vi "Calc Arc Angles.vi"(10 "Arc CMD":T1={"N"=0.0, "GCODE"="", "X"=2.0396, "Y"=0.1665, "Z"=0.0, "E"=0.0, "I"=0.205, "J"=0.131, "S"=0.0, "F"=0.0}, 11 "Initial CMD":T1={"N"=0.0, "GCODE"="", "X"=1.6296, "Y"=0.1665, "Z"=-0.05, "E"=0.0, "I"=0.0, "J"=0.0, "S"=0.0, "F"=0.0}) -> (0 "travel angle out":dbl=114.84085989051317 format="%.5f", 2 "start angle (tangent)":dbl=212.57957005474344 format="%#_8g", 3 "R":dbl=0.2432817296880306 format="%#_9g")   [LabVIEW 2014]
uses:
  GCode Parser/GCode Command Cluster.ctl
panel:
  out "x*y":dbl=32.57957005474343
  out "V2Y":dbl=-0.13099999999999998
  out "V2X":dbl=0.20500000000000007
  out "V1Y":dbl=-0.13099999999999998
  out "V1X":dbl=-0.20500000000000007
  out "theta (degrees)":dbl=-114.84085989051317 format="%.2f"
  out "theta (radians)":dbl=-2.0043511209109495 format="%.3f"
  # "G01 X1.6296 Y0.1665 Z-0.0500\nG03 X2.0396 Y0.1665 I0.2050 J0.1310"
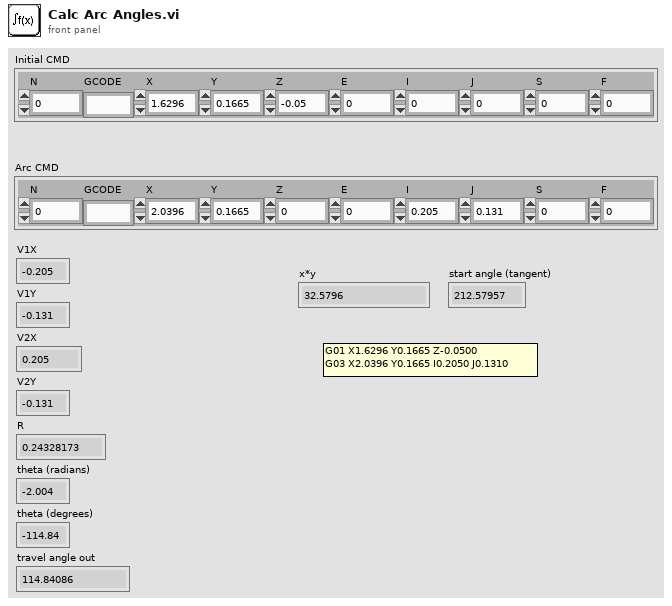
[diagram p1: front panel]
types:
  T1 = typedef "GCode Command Cluster.ctl" = cluster{"N":dbl, "GCODE":string, "X":dbl, "Y":dbl, "Z":dbl, "E":dbl, "I":dbl, "J":dbl, "S":dbl, "F":dbl}
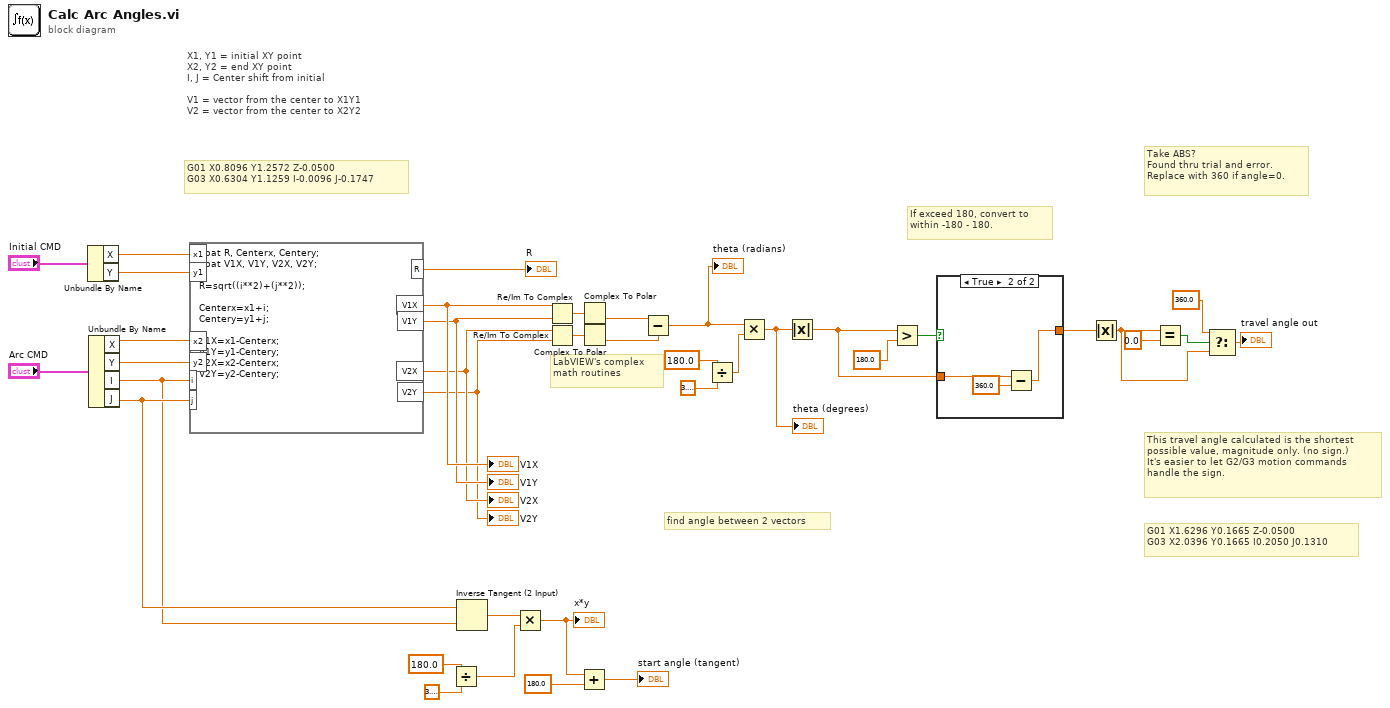
[diagram p0: block diagram]
diagram:
  # "This travel angle calculated is the shortest\npossible value, magnitude only. (no sign.)\nIt's easier to let G2/G3 motion commands\nhandle the sign."
  # "If exceed 180, convert to \nwithin -180 - 180."
  # "G01 X1.6296 Y0.1665 Z-0.0500\nG03 X2.0396 Y0.1665 I0.2050 J0.1310"
  # "Take ABS?\nFound thru trial and error.\nReplace with 360 if angle=0."
  # "find angle between 2 vectors"
  # "X1, Y1 = initial XY point\nX2, Y2 = end XY point\nI, J = Center shift from initial \n\nV1 = vector from the center to X1Y1\nV2 = vector from the center to X2Y2"
  # "LabVIEW's complex\nmath routines"
  # "G01 X0.8096 Y1.2572 Z-0.0500\nG03 X0.6304 Y1.1259 I-0.0096 J-0.1747"
  n1 = Unbundle By Name("Initial CMD") -> ("X"=w18:dbl, "Y"=w19:dbl)
  n2 = Unbundle By Name("Arc CMD") -> ("X"=w17:dbl, "Y"=w16:dbl, "I"=w14:dbl, "J"=w15:dbl)
  n3 = formula code="float R, Centerx, Centery;\nfloat V1X, V1Y, V2X, V2Y;\n\nR=sqrt((i**2)+(j**2));\n\nCenterx=x1+i;\nCentery=y1+j;\n\nV1X=x1-Centerx;\nV1Y=y1-Centery;\nV2X=x2-Centerx;\nV2Y=y2-Centery;"("x2"=w17, "x1"=w18, "y2"=w16, "y1"=w19, "i"=w14, "j"=w15) -> ("R"=→"R":dbl, "V1X"=w29:dbl, "V1Y"=w28:dbl, "V2X"=w27:dbl, "V2Y"=w26:dbl)
  "V1X" <- w29
  "V1Y" <- w28
  "V2X" <- w27
  "V2Y" <- w26
  n4 = Divide(x=180.0, y=3.141592653589793) -> (x/y=w11:dbl)
  n5 = Inverse Tangent (2 Input)(1:w14, 2:w15) -> (0:w10:dbl)
  n6 = Multiply(x=w10, y=w11) -> (x*y=w6:dbl)
  "x*y" <- w6
  n7 = Re/Im To Complex(1:w28, 2:w29) -> (0:w37:cdb)
  n8 = Re/Im To Complex(1:w26, 2:w27) -> (0:w36:cdb)
  n9 = Add(x=w6, y=180.0) -> (x+y=→"start angle (tangent)":dbl)
  n10 = Complex To Polar(r * e^(i*theta)=w37) -> (theta=w32:dbl)  [unwired: 1 out]
  n11 = Complex To Polar(r * e^(i*theta)=w36) -> (theta=w31:dbl)  [unwired: 1 out]
  n12 = Subtract(x=w32, y=w31) -> (x-y=w33:dbl)
  "theta (radians)" <- w33
  n13 = Divide(x=180.0, y=3.141592653589793) -> (x/y=w30:dbl)
  n14 = Multiply(x=w33, y=w30) -> (x*y=w4:dbl)
  "theta (degrees)" <- w4
  n15 = Absolute Value(x=w4) -> (abs(x)=w2:dbl)
  n16 = Greater?(x=w2, y=180.0) -> (0:w1:bool)
  n17 = case shown="True" w1 {
    tunnel: w2 -> [w39 w42]
    tunnel: [w39 w40] -> w5
    frame False {
    }
    frame True {
      n18 = Subtract(x=w42, y=360.0) -> (x-y=w40:dbl)
    }
  }
  n19 = Absolute Value(x=w5) -> (abs(x)=w9:dbl)
  n20 = Equal?(x=w9, y=0.0) -> (x = y?=w25:bool)
  n21 = Select(t=360.0, s=w25, f=w9) -> (s? t:f=→"travel angle out":dbl)
